vi "Main Tree _ Initialize.vi"(8 "error in":errorcluster caption="错误输入", 11 "Ref.Tree Ref":refnum<vi>) -> (0 "error out":errorcluster caption="错误输出")   [LabVIEW 2016]
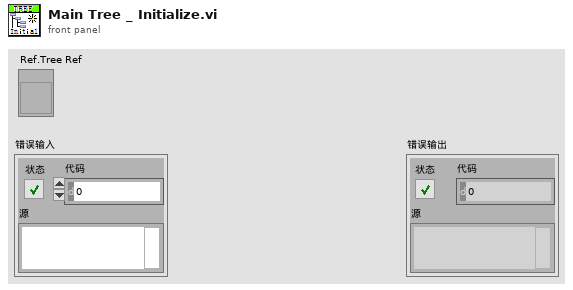
[diagram p1: front panel]
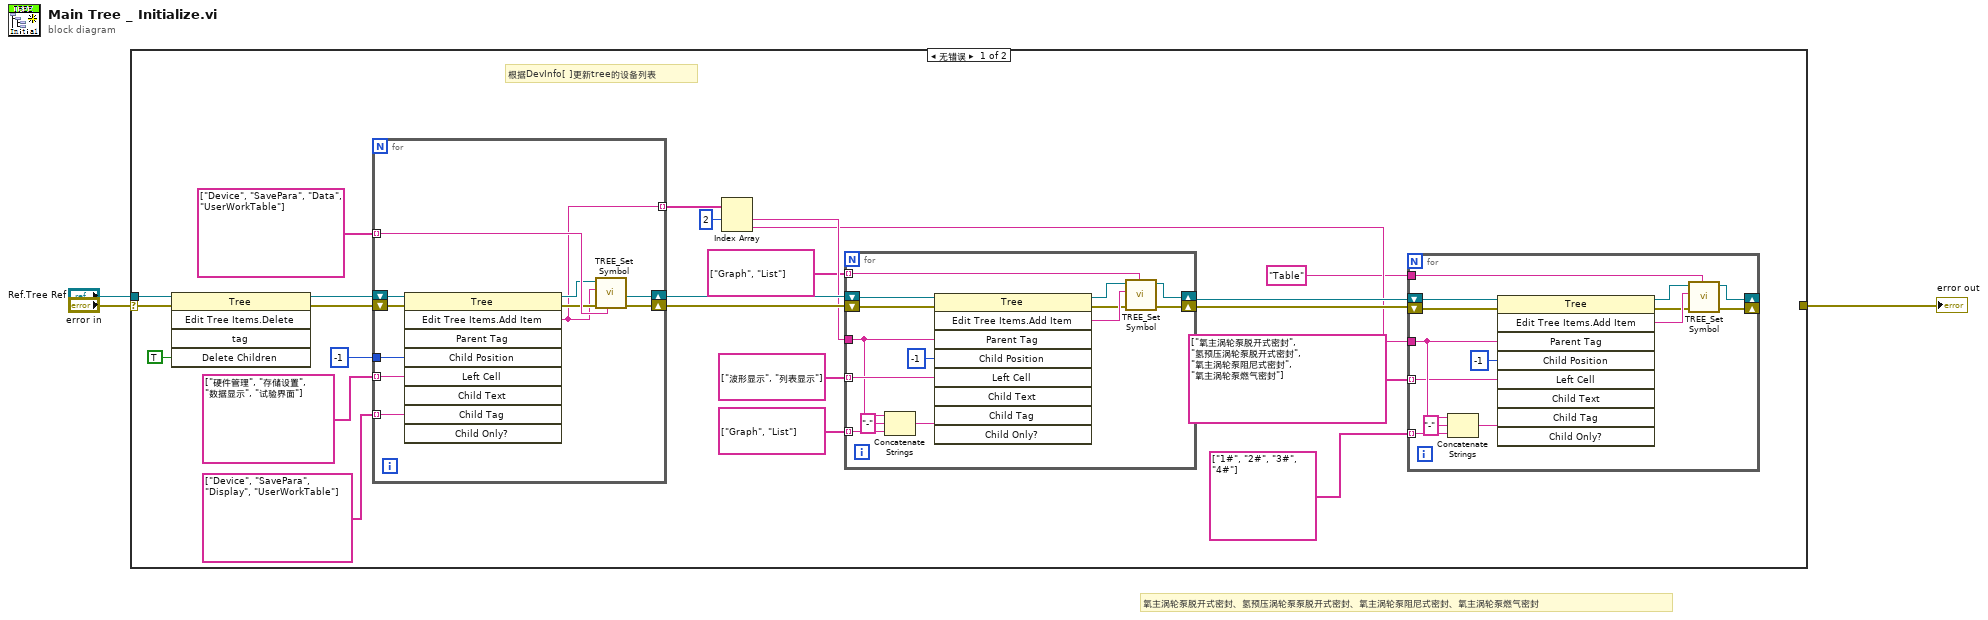
[diagram p0: block diagram]
diagram:
  # "氧主涡轮泵脱开式密封、氢预压涡轮泵泵脱开式密封、氧主涡轮泵阻尼式密封、氧主涡轮泵燃气密封"
  n1 = case shown="无错误" "error in" {
    selector: "error in" -> [w25 w66]
    tunnel: [_ w66] -> w2
    tunnel: "Ref.Tree Ref" -> [w26 _]
    frame No Error {
      # "根据DevInfo[ ]更新tree的设备列表"
      n2 = invoke class="Tree" method="Edit Tree Items.Delete"(reference=w26, error in=w25, "Delete Children"=TRUE ("删除子项？")) -> (reference out=w23:refnum<vi>, error out=w22:errorcluster)  [unwired: 2 in, 3 out]
      n3 = for {
        tunnel: string[] ["Device", "SavePara", "Data", "UserWorkTable"] -> [w51] mode=indexing
        tunnel: string[] ["硬件管理", "存储设置", "数据显示", "试验界面"] -> [w48] mode=indexing
        tunnel: string[] ["Device", "SavePara", "Display", "UserWorkTable"] -> [w47] mode=indexing
        tunnel: -1 ("子项位置") -> [w42]
        shift-right: [w43] -> w19
        shift-left: w23 -> [w50]
        shift-right: [w44] -> w20
        shift-left: w22 -> [w49]
        tunnel: [w41] -> w11 mode=indexing
        n4 = invoke class="Tree" method="Edit Tree Items.Add Item"(reference=w50, error in=w49, "Child Position"=w42, "Left Cell"=w48, "Child Tag"=w47) -> (reference out=w46:refnum<vi>, error out=w45:errorcluster, "Edit Tree Items:Add Item"=w41:string)  [unwired: 4 in, 6 out]
        n5 = call "TREE_Set Symbol.vi"("PicName"=w51, "error in"=w45, "Tag"=w41, "Tree Ref"=w46) -> ("error out"=w44:errorcluster, "Tree Ref"=w43:refnum<vi>)  [unwired: 6 in]
      }
      n6 = Index Array(array=w11, index #1=2 ("index")) -> (element #1=w17:string, element #2=w7:string)  [unwired: 1 in]
      n7 = for {
        shift-right: [w59] -> w8
        shift-left: w19 -> [w60]
        shift-right: [w58] -> w9
        shift-left: w20 -> [w61]
        tunnel: string[] ["波形显示", "列表显示"] -> [w57] mode=indexing
        tunnel: w17 -> [w56]
        tunnel: string[] ["Graph", "List"] -> [w54] mode=indexing
        tunnel: string[] ["Graph", "List"] -> [w52] mode=indexing
        n8 = Concatenate Strings(w56, "-" ("字符串"), w54) -> (w55:string)
        n9 = invoke class="Tree" method="Edit Tree Items.Add Item"(reference=w60, error in=w61, "Parent Tag"=w56, "Child Position"=-1 ("子项位置"), "Left Cell"=w57, "Child Tag"=w55) -> (reference out=w63:refnum<vi>, error out=w62:errorcluster, "Edit Tree Items:Add Item"=w64:string)  [unwired: 3 in, 6 out]
        n10 = call "TREE_Set Symbol.vi"("PicName"=w52, "error in"=w62, "Tag"=w64, "Tree Ref"=w63) -> ("error out"=w58:errorcluster, "Tree Ref"=w59:refnum<vi>)  [unwired: 6 in]
      }
      n11 = for {
        shift-right: [w34] -> _
        shift-left: w8 -> [w35]
        shift-right: [w33] -> _
        shift-left: w9 -> [w36]
        tunnel: string[] ["氧主涡轮泵脱开式密封", "氢预压涡轮泵脱开式密封", "氧主涡轮泵阻尼式密封", "氧主涡轮泵燃气密封"] -> [w27] mode=indexing
        tunnel: w7 -> [w32]
        tunnel: string[] ["1#", "2#", "3#", "4#"] -> [w30] mode=indexing
        tunnel: "Table" -> [w28]
        n12 = Concatenate Strings(w32, "-" ("字符串"), w30) -> (w31:string)
        n13 = invoke class="Tree" method="Edit Tree Items.Add Item"(reference=w35, error in=w36, "Parent Tag"=w32, "Child Position"=-1 ("子项位置"), "Left Cell"=w27, "Child Tag"=w31) -> (reference out=w38:refnum<vi>, error out=w37:errorcluster, "Edit Tree Items:Add Item"=w39:string)  [unwired: 3 in, 6 out]
        n14 = call "TREE_Set Symbol.vi"("PicName"=w28, "error in"=w37, "Tag"=w39, "Tree Ref"=w38) -> ("error out"=w33:errorcluster, "Tree Ref"=w34:refnum<vi>)  [unwired: 6 in]
      }
    }
    frame Error {
    }
  }
  "error out" <- w2
